vi "Write CPC Data.vi"(8 "error in (no error)":errorcluster, 10 "CPC Data":refnum<class "CPC Data.lvclass">, 11 "CPC in":refnum<class "CPC.lvclass">) -> (0 "error out":errorcluster, 3 "CPC out":refnum<class "CPC.lvclass">)   [LabVIEW 2013, in "CPC.lvclass"]
uses:
  CPC.lvclass
  CPC Data.lvclass
  CPC.lvclass/CPC.ctl
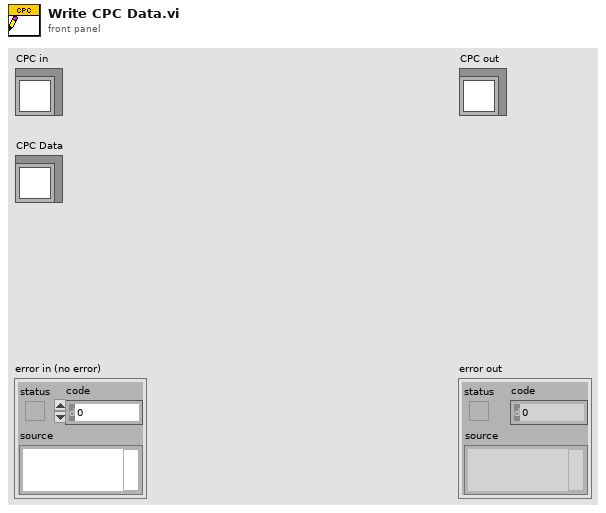
[diagram p1: front panel]
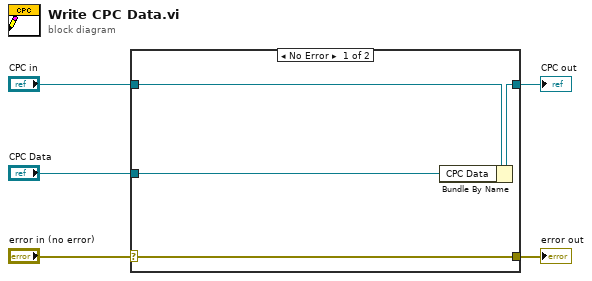
[diagram p0: block diagram]
diagram:
  n1 = case shown="No Error" "error in (no error)" {
    selector: "error in (no error)" -> [w9 w10]
    tunnel: [w9 w10] -> w4
    tunnel: [w7 w11] -> w2
    tunnel: "CPC in" -> [w8 w11]
    tunnel: "CPC Data" -> [w6 _]
    frame No Error {
      n2 = Bundle By Name(cluster=w8, "CPC Data"=w6) -> (w7:refnum<class "CPC.lvclass">)
    }
    frame Error {
    }
  }
  "error out" <- w4
  "CPC out" <- w2
